vi "Stopped.vi"(6 "Teller":T1 {"AbsoluteTime" format="%<%x %.3X>T"}, 8 "Error in":errorcluster, 9 "Error":errorcluster, 10 "Actor":refnum<class "Actor.lvclass">, 11 "Base Actor in":refnum<class "Base Actor.lvclass">) -> (0 "Error out":errorcluster, 3 "Base Actor out":refnum<class "Base Actor.lvclass">)   [LabVIEW 2020, in "jettl.lvlib" / "BaseActor.lvlib" / "Base Actor.lvclass"]
uses:
  Base Actor.lvclass
  Base Actor.lvclass/Base Actor.ctl
  Actor/Actor.lvclass
  jettl.lvlib
  ActorLifetime.ctl
  ActorRelation.ctl
  MessageMetadata.ctl
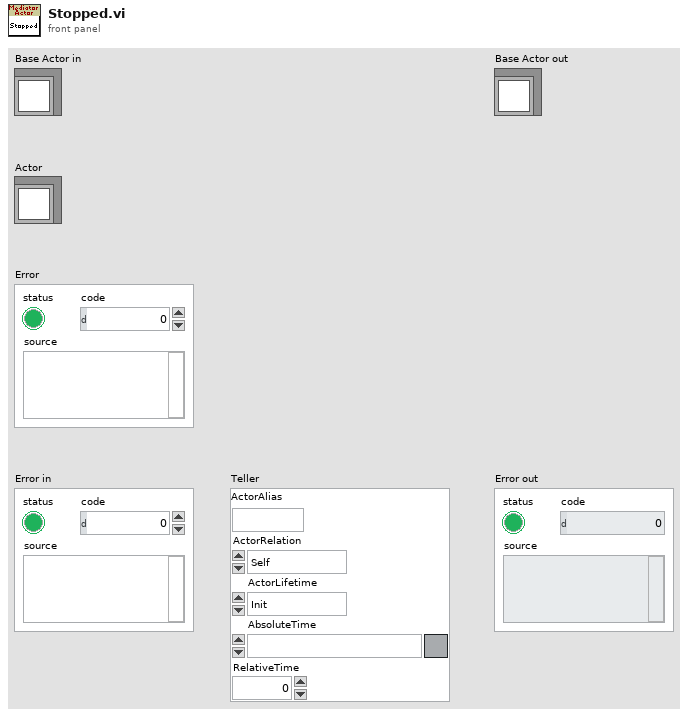
[diagram p1: front panel]
types:
  T1 = typedef "jettl.lvlib/MessageMetadata.ctl" = cluster{"ActorAlias":string, "ActorRelation":T2, "ActorLifetime":T3, "AbsoluteTime":timestamp, "RelativeTime":dbl}
  T2 = typedef "jettl.lvlib/ActorRelation.ctl" = enum16{"Self", "Mediator", "Component"}
  T3 = typedef "jettl.lvlib/ActorLifetime.ctl" = enum16{"Init", "Spawn", "Setup", "Teardown Before Running", "Running", "Stop Called", "Stopping With Children", "Stopping Without Children", "Teardown After Running", "Stopped"}
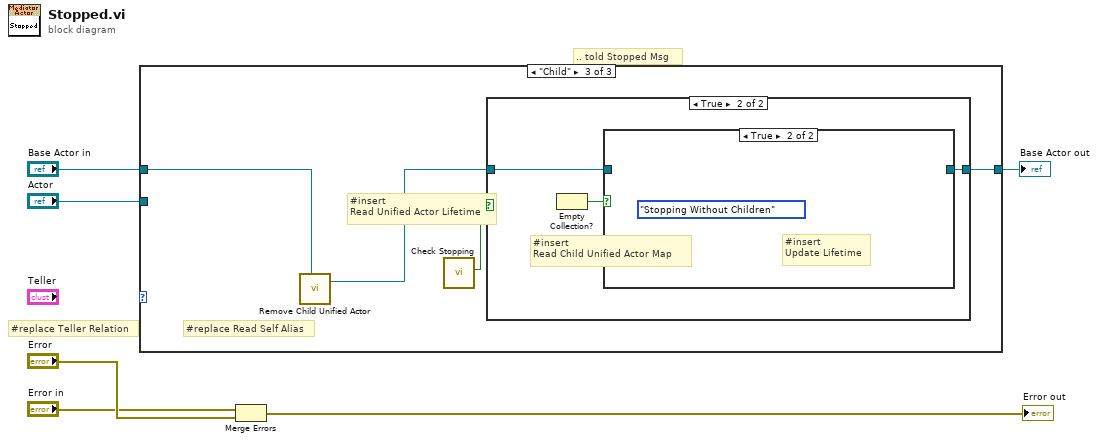
[diagram p0: block diagram]
diagram:
  # "#replace Teller Relation"
  # ".. told Stopped Msg"
  n1 = case shown="\"Child\"" {
    selector: _ -> [_ _ _]
    tunnel: "Base Actor in" -> [w7 w8 w10]
    tunnel: [w7 w8 w12] -> w6
    tunnel: "Actor" -> [_ _ w11]
    frame "Self" {
      # "Case will not fundamentally execute"
    }
    frame "Parent" {
      # "Case will not fundamentally execute"
    }
    frame "Child" {
      # "#insert\nRead Unified Actor Lifetime"
      # "#replace Read Self Alias"
      n2 = call "Remove Child Unified Actor.vi"("Actor in"=w10) -> ("Actor out"=w9:refnum<class "Actor.lvclass">)  [unwired: 10 in]
      n3 = call "Check Stopping.vi"() -> ("Stopping"=w13:bool)  [unwired: 11 in]
      n4 = case shown="True" w13 {
        tunnel: w9 -> [w14 w15]
        tunnel: [w14 w17] -> w12
        frame False {
        }
        frame True {
          # "#insert\nRead Child Unified Actor Map"
          n5 = Empty Collection?() -> (0:w16:bool)  [unwired: 1 in]
          n6 = case shown="True" w16 {
            tunnel: [w18 w19] -> w17
            tunnel: w15 -> [w18 w20]
            frame False {
            }
            frame True {
              w21 = ActorLifetime."Stopping Without Children" ("Lifetime")
              # "#insert\nUpdate Lifetime"
            }
          }
        }
      }
    }
  }
  "Base Actor out" <- w6
  n7 = Merge Errors("Error in", "Error") -> (→"Error out":errorcluster)
